vi "FisherPaykel Set Current Limit.vi"(7 "Debug":bool, 8 "Error In":errorcluster, 9 "Current Limit - (1-50) - (0.1-5A)":u16 max=50 step=1, 10 "Main Command":T1=">PA", 11 "VISA Refnum in":refnum<visa-resource-name>) -> (0 "Error Out":errorcluster, 3 "VISA Refnum out":refnum<visa-resource-name>)   [LabVIEW 2016]
uses:
  Type Definitions/Fisher Paykel Main Command.ctl
panel:
  out "Command (Debug)":string
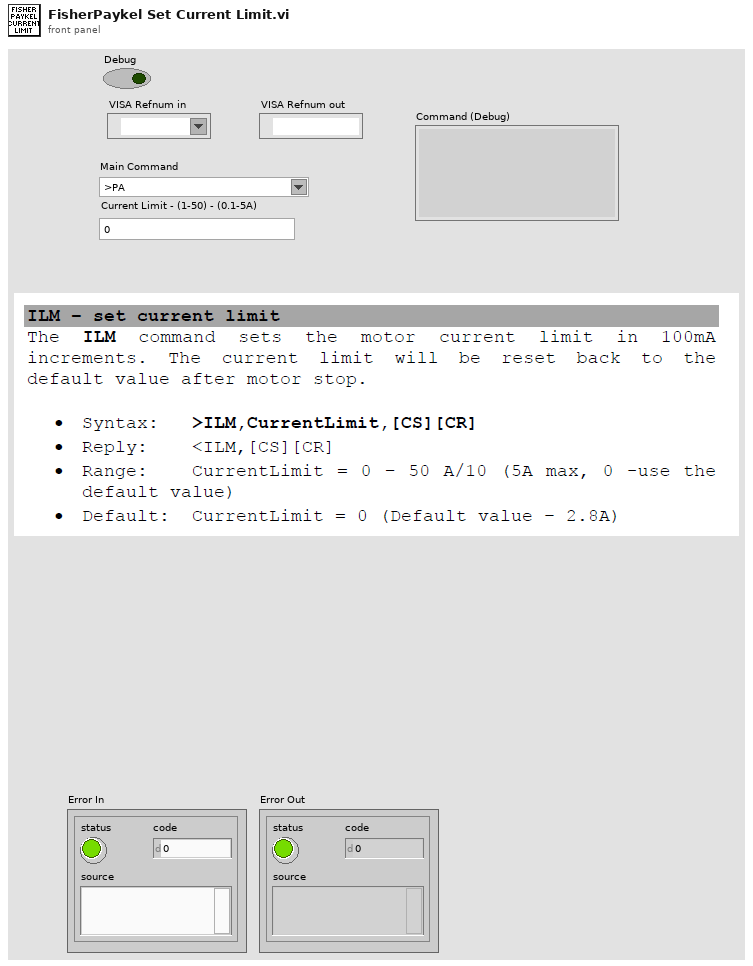
[diagram p1: front panel]
types:
  T1 = typedef "Fisher Paykel Main Command.ctl" = string
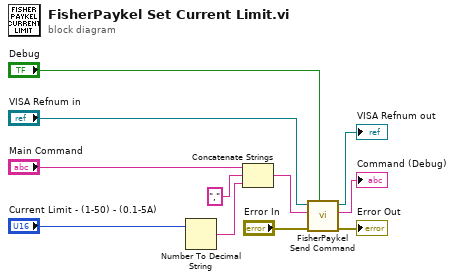
[diagram p0: block diagram]
diagram:
  n1 = Number To Decimal String(number="Current Limit - (1-50) - (0.1-5A)") -> (decimal integer string=w1:string)  [unwired: 1 in]
  n2 = Concatenate Strings("Main Command", ",", w1) -> (w5:string)
  n3 = call "FisherPaykel Send Command.vi"("Debug"="Debug", "error in (no error)"="Error In", "Send Command"=w5, "VISA Refnum in"="VISA Refnum in") -> ("error out"=→"Error Out":errorcluster, "Command (Debug)"=→"Command (Debug)":string, "VISA Refnum out"=→"VISA Refnum out":refnum<visa-resource-name>)  [unwired: 5 in]
